vi "Anritsu VNA Read Trace Display.vi"(4 "Trace":i8=1 min=1 max=99 step=1, 6 "Channel":i8=1 min=1 max=99 step=1, 7 "Anritsu VNA":T1, 8 "error in (no error)":errorcluster, 11 "VISA Resource Name":refnum<visa-resource-name>) -> (0 "error out":errorcluster, 2 "Displayed?":bool, 3 "dup VISA Resource Name":refnum<visa-resource-name>)   [LabVIEW 2011]
uses:
  TypeDefs/Anritsu VNA Instrument Info.ctl
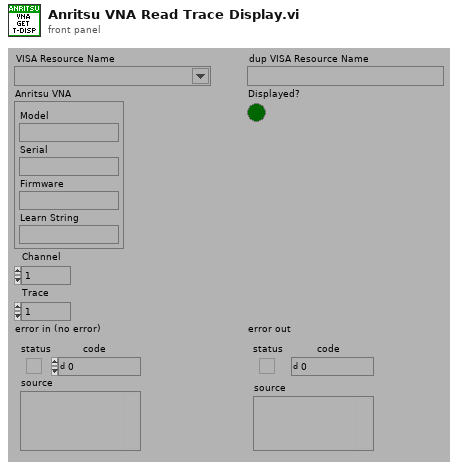
[diagram p1: front panel]
types:
  T1 = typedef "Anritsu VNA Instrument Info.ctl" = cluster{"Model":string, "Serial":string, "Firmware":string, "Learn String":string}
  T2 = typedef "Anritsu VNA Model.ctl" = enum16{"Not Supported", "37XXXX", "MS20XXX", "MS462XX", "MS464XX"}
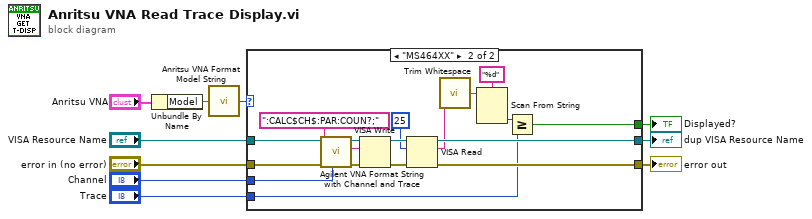
[diagram p0: block diagram]
diagram:
  n1 = Unbundle By Name("Anritsu VNA") -> ("Model"=w1:string)
  n2 = call "Anritsu VNA Format Model String.vi"("Model"=w1) -> ("Model"=w6:T2)
  n3 = case shown="\"MS464XX\"" w6 {
    tunnel: "VISA Resource Name" -> [w12 w28]
    tunnel: "error in (no error)" -> [w11 w27]
    tunnel: [w12 w24] -> w8
    tunnel: [w11 w23] -> w7
    tunnel: [_ w13] -> w5
    tunnel: "Channel" -> [_ w18]
    tunnel: "Trace" -> [_ w14]
    frame "Not Supported".."MS462XX" {
    }
    frame "MS464XX" {
      n4 = call "Agilent VNA Format String with Channel and Trace.vi"("Channel"=w18, "String"=":CALC$CH$:PAR:COUN?;" ("write buffer")) -> ("String Out"=w19:string)  [unwired: 1 in, 6 out]
      n5 = VISA Write(VISA resource name=w28, write buffer=w19, error in (no error)=w27) -> (VISA resource name out=w25:refnum<visa-resource-name>, error out=w26:errorcluster)  [unwired: 1 out]
      n6 = VISA Read(VISA resource name=w25, byte count=u32 25, error in (no error)=w26) -> (VISA resource name out=w24:refnum<visa-resource-name>, read buffer=w21:string, error out=w23:errorcluster)  [unwired: 1 out]
      n7 = call <vilib>:"Trim Whitespace.vi"("string"=w21) -> ("trimmed string"=w17:string)  [unwired: 1 in]
      n8 = Scan From String(format string="%d", input string=w17) -> (output 1=w15:i32)  [unwired: 2 in, 4 out]
      n9 = Greater Or Equal?(x=w15, y=w14) -> (x >= y?=w13:bool)
    }
  }
  "dup VISA Resource Name" <- w8
  "error out" <- w7
  "Displayed?" <- w5
